vi "Read Collected Data2D.vi"(8 "error in (no error)":errorcluster, 11 "AbstractCollector2D in":refnum<class "AbstractCollector2D.lvclass">) -> (0 "error out":errorcluster, 2 "Collected Data":refnum<class "Data2D.lvclass">, 3 "AbstractCollector2D out":refnum<class "AbstractCollector2D.lvclass">)   [LabVIEW 2014, in "AbstractCollector2D.lvclass"]
uses:
  AbstractCollector2D.lvclass
  Model/Data/Data2D/Data2D.lvclass
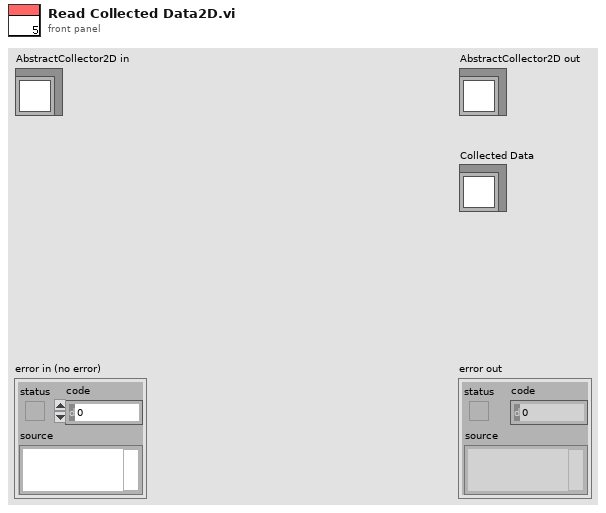
[diagram p1: front panel]
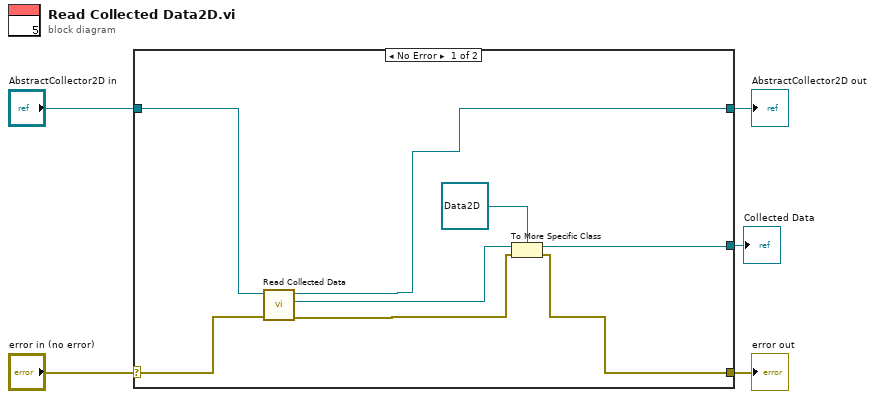
[diagram p0: block diagram]
diagram:
  n1 = case shown="No Error" "error in (no error)" {
    selector: "error in (no error)" -> [w11 w15]
    tunnel: [w10 w15] -> w4
    tunnel: [w8 w14] -> w2
    tunnel: "AbstractCollector2D in" -> [w9 w14]
    tunnel: [w6 _] -> w1
    frame No Error {
      n2 = call-dynamic "Read Collected Data.vi"("error in (no error)"=w11, "AbstractCollector in"=w9) -> ("error out"=w13:errorcluster, "Collected Data"=w12:refnum<class "AbstractData.lvclass">, "AbstractCollector out"=w8:refnum<class "AbstractCollector2D.lvclass">)  [unwired: 7 in]
      n3 = To More Specific Class(target class=refnum<class "Data2D.lvclass"> refnum ("Data2D.lvclass"), reference=w12, error in=w13) -> (specific class reference=w6:refnum<class "Data2D.lvclass">, error out=w10:errorcluster)
    }
    frame Error {
    }
  }
  "error out" <- w4
  "AbstractCollector2D out" <- w2
  "Collected Data" <- w1
